vi "ATF Storage-waveform Samples bulider.vi"(7 "Samples":i32=10, 9 "Data input":waveform(dbl)[](array[waveform]), 11 "AI_C_Data RD":refnum<queue>) -> (1 "Data out":waveform(dbl)[](array[waveform]))   [LabVIEW 2022 SP3]
panel:
  out "overflow?":bool
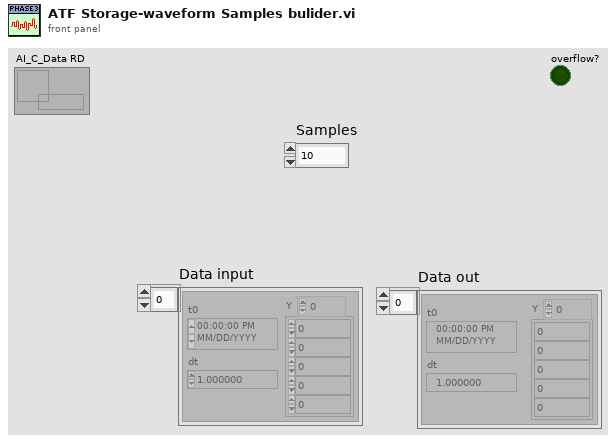
[diagram p1: front panel]
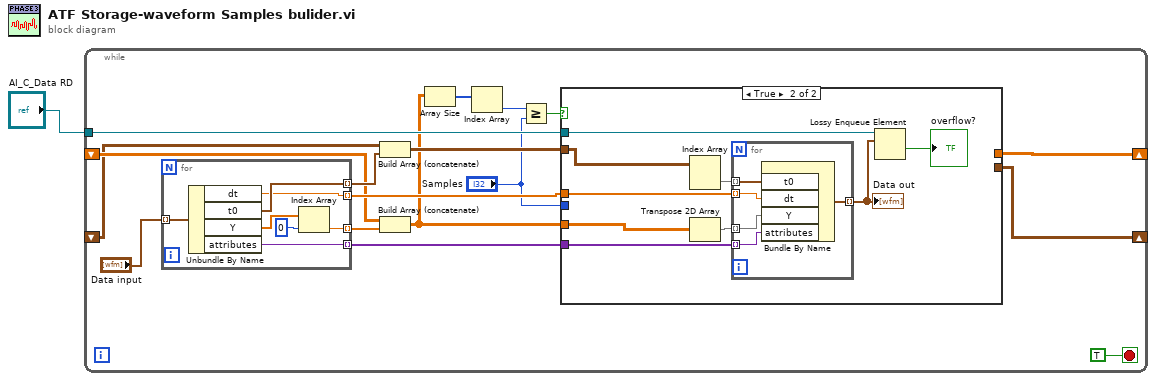
[diagram p0: block diagram]
diagram:
  n1 = while {
    tunnel: "AI_C_Data RD" -> [w18]
    shift-right: [w5] -> _
    shift-left: _ -> [w4]
    shift-right: [w6] -> _
    shift-left: _ -> [w3]
    stop <- TRUE stop-if-true
    n2 = for {
      tunnel: "Data input" -> [w41] mode=indexing
      tunnel: [w39] -> w8 mode=indexing
      tunnel: [w37] -> w14 mode=indexing
      tunnel: [w36] -> w16 mode=indexing
      tunnel: [w35] -> w17 mode=indexing
      n3 = Unbundle By Name(w41) -> ("dt"=w35:dbl, "t0"=w37:timestamp, "Y"=w40:dbl[], "attributes"=w36:variant)
      n4 = Index Array(array=w40, index=0) -> (element=w39:dbl)
    }
    n5 = Build Array (concatenate)(w3, w14) -> (w15:timestamp[][])
    n6 = Build Array (concatenate)(w4, w8) -> (w11:dbl[][])
    n7 = Array Size(array=w11) -> (size(s)=w9:i32[])
    n8 = Index Array(array=w9) -> (element=w10:i32)  [unwired: 1 in]
    n9 = Greater Or Equal?(x=w10, y="Samples") -> (x >= y?=w12:bool)
    n10 = case shown="True" w12 {
      tunnel: w11 -> [w20 w21]
      tunnel: [w20 _] -> w5
      tunnel: w15 -> [w19 w29]
      tunnel: [w19 _] -> w6
      tunnel: w16 -> [_ w27]
      tunnel: w17 -> [_ w25]
      tunnel: "Samples" -> [_ _]
      tunnel: w18 -> [_ w24]
      frame False {
      }
      frame True {
        n11 = Index Array(array=w29) -> (element=w28:timestamp[])  [unwired: 2 in]
        n12 = Transpose 2D Array(2D array=w21) -> (transposed array=w26:dbl[][])
        n13 = for {
          tunnel: w26 -> [w34] mode=indexing
          tunnel: w28 -> [w33] mode=indexing
          tunnel: w27 -> [w32] mode=indexing
          tunnel: [w31] -> w23 mode=indexing
          tunnel: w25 -> [w30] mode=indexing
          n14 = Bundle By Name("t0"=w33, "dt"=w30, "Y"=w34, "attributes"=w32) -> (w31:waveform(dbl))  [unwired: 1 in]
        }
        "Data out" <- w23
        n15 = Lossy Enqueue Element(queue=w24, element=w23) -> (overflow?=→"overflow?":bool)  [unwired: 1 in, 3 out]
      }
    }
  }
